vi "Initialize Sink.vi"(11 "String Control Sink in":refnum<class "String Control Sink.lvclass">) -> (0 "error out":errorcluster, 3 "String Control Sink out":refnum<class "String Control Sink.lvclass">)   [LabVIEW 2020, in "String Control Sink.lvclass"]
uses:
  <vilib>/gpm_packages/@cs/event-logger/Source/String Control Sink/String Control Sink.lvclass
  <vilib>/gpm_packages/@cs/event-logger/Source/String Control Sink/String Control Sink.lvclass/String Control Sink.ctl
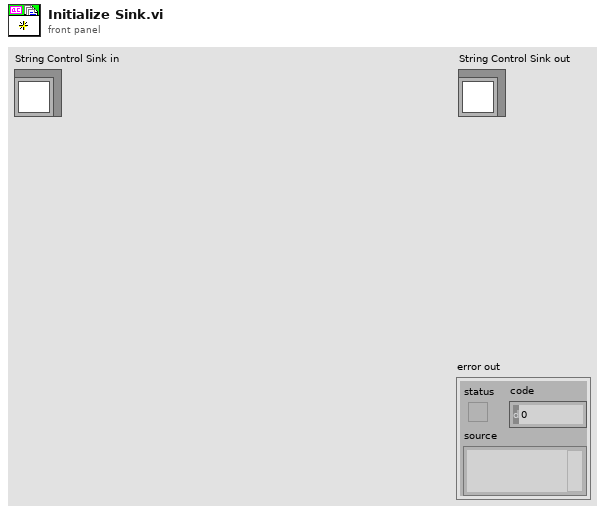
[diagram p1: front panel]
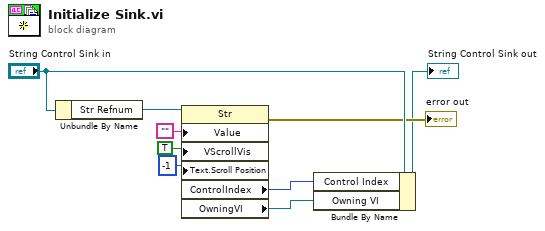
[diagram p0: block diagram]
diagram:
  n1 = Unbundle By Name("String Control Sink in") -> ("Str Refnum"=w9:refnum<vi>)
  n2 = property class="Str"(reference=w9, "Value"="", "VScrollVis"=TRUE ("Vertical Scrollbar Visible"), "Text.Scroll Position"=-1) -> (error out=→"error out":errorcluster, "ControlIndex"=w2:i32, "OwningVI"=w1:refnum<vi>)  [unwired: 1 in, 1 out]
  n3 = Bundle By Name(cluster="String Control Sink in", "Control Index"=w2, "Owning VI"=w1) -> (→"String Control Sink out":refnum<class "String Control Sink.lvclass">)
